vi "ReadUSB.vi"() -> ()   [LabVIEW 2018]
uses:
  <vilib>/Instr/_visa.llb/VISA Configure Serial Port (Instr).vi
panel:
  in  "ch":bool
  out "Erro de estado estacionário":dbl=3.0 format="%#_13g"
  out "Máximo Overshoot":dbl=3.0 format="%#_13g"
  out "Tempo de Subida":dbl=3.0 format="%#_13g"
  out "Tempo de Acomodação":dbl=3.0 format="%#_13g"
  in  "Modo Simulação":bool
  in  "Tempo de Simulação":dbl=3.0 format="%#_13g"
  out "cmd":T1(ring)
  in  "graph index":i32
  in  "Motor":cluster{"2":bool, "3":bool, "0":bool, "1":bool}={"2"=TRUE, "3"=FALSE, "0"=FALSE, "1"=FALSE}
  in  "Write":T2={"get_vel"=TRUE, "set_vel"=FALSE, "get PID cte"=FALSE, "set PID cte"=FALSE}
  out "String Enviada":string
  in  "kd":dbl format="%#_13g"
  in  "ki":dbl format="%#_13g"
  in  "kp":dbl format="%#_13g"
  in  "Vel":dbl format="%#_13g"
  out "kd":dbl
  out "ki":dbl
  out "kp":dbl
  out "String Tratada":string
  out "String Lida":string
  out "Vel":dbl
  in  "End":bool
  out "config error":errorcluster
  out "Vel":cluster{dbl, " Vel":dbl}(graph)
  in  "VISA resource name":refnum<visa-resource-name>
  # "APERTE END PARA ENCERRAR O PROGRAMA"
  # "VSS"
  # "SSL"
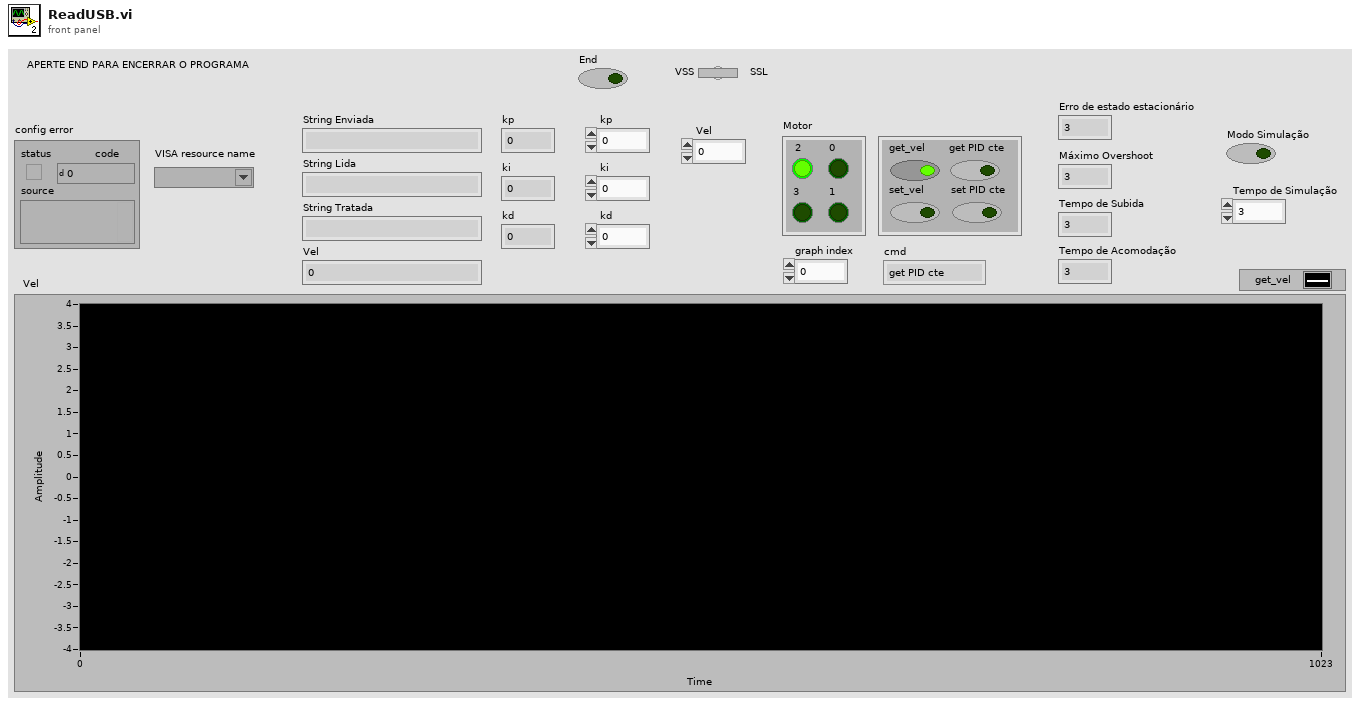
[diagram p1: front panel]
types:
  T1 = enum16{"get PID cte", "Set Vel", "Set PID cte", "get Vel"}
  T2 = cluster{"get_vel":bool, "set_vel":bool, "get PID cte":bool, "set PID cte":bool}
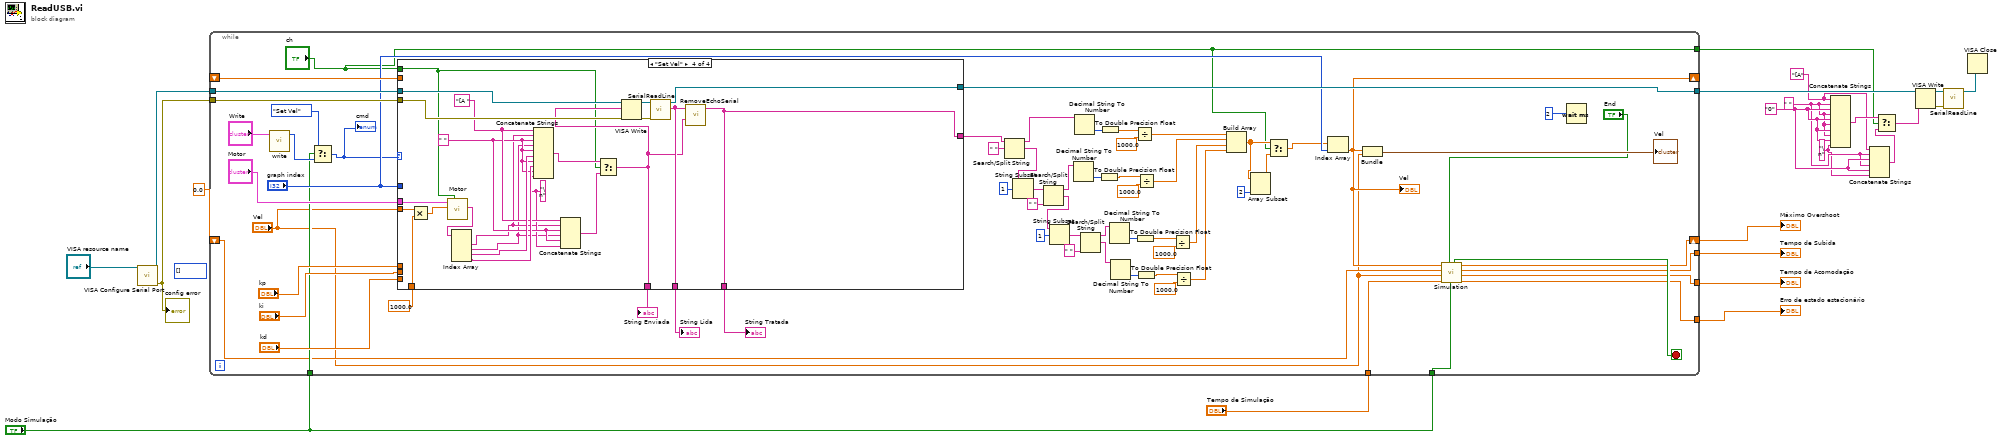
[diagram p0: block diagram]
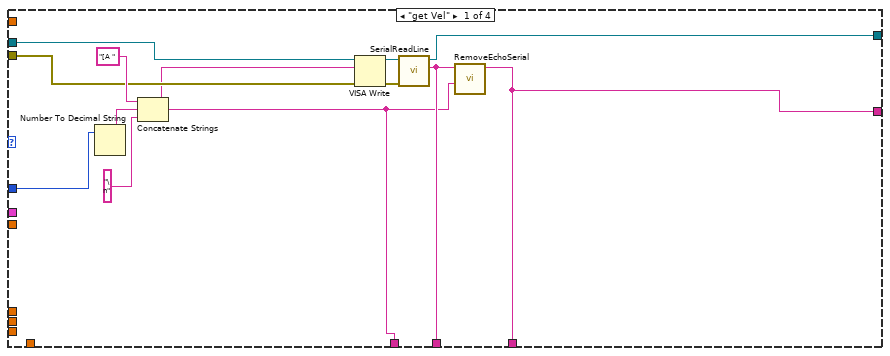
[diagram p2: hidden frame]
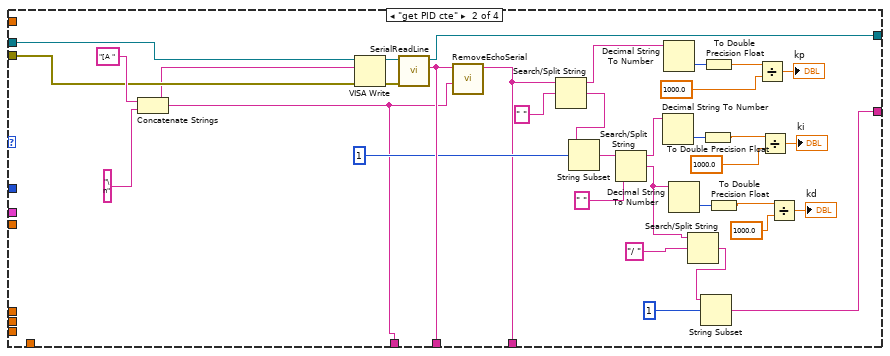
[diagram p3: hidden frame]
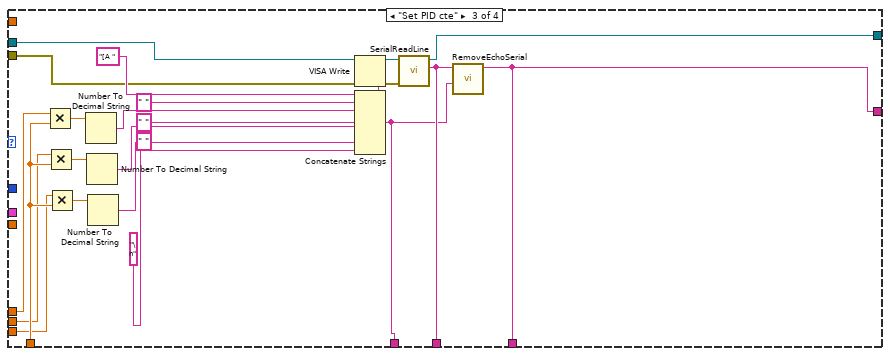
[diagram p4: hidden frame]
diagram:
  w2 = "\n" ("string")
  w4 = "0" ("string")
  w3 = " " ("string")
  w5 = "[A" ("write buffer")
  (unwired) i32[] []
  n1 = call-poly "VISA Configure Serial Port"("VISA resource name"="VISA resource name") -> ("VISA resource name out"=w20:refnum<visa-resource-name>, "error out"=w21:errorcluster)  [unwired: 13 in]
  "config error" <- w21
  n2 = while {
    tunnel: w21 -> [w87]
    tunnel: w20 -> [w86]
    tunnel: [w85] -> w16
    shift-right: [w31] -> _
    shift-left: _ -> [w82]
    tunnel: "Tempo de Simulação" -> [w42]
    tunnel: "Modo Simulação" -> [w39]
    tunnel: "Modo Simulação" -> [w37]
    shift-right: [w34] -> w12
    shift-left: 0.0 -> [w33]
    tunnel: [w32] -> w11
    tunnel: [w29] -> w10
    tunnel: [w28] -> w9
    tunnel: ["ch"] -> w7
    stop <- w40 stop-if-true
    n3 = call "write.vi"("Write"="Write") -> ("s? t:f"=w38:T1)  [unwired: 10 in]
    n4 = Select(t=T1."Set Vel", s=w37, f=w38) -> (s? t:f=w35:T1)
    "cmd" <- w35
    n5 = case shown="\"Set Vel\"" w35 {
      tunnel: w87 -> [w95 w129 w154 w178]
      tunnel: w86 -> [w94 w128 w153 w177]
      tunnel: [w93 w127 w152 w176] -> w85
      tunnel: "graph index" -> [w91 _ _ _]
      tunnel: [w92 w126 w151 w175] -> w84
      tunnel: [w90 w124 w136 w172] -> w83
      tunnel: w82 -> [_ _ _ _]
      tunnel: "Vel" -> [_ _ _ w174]
      tunnel: 1000.0 -> [_ _ w145 w173]
      tunnel: "kp" -> [_ _ w144 _]
      tunnel: "ki" -> [_ _ w143 _]
      tunnel: "kd" -> [_ _ w142 _]
      tunnel: [w90 w102 w136 w172] -> w48
      tunnel: [w89 w101 w135 w159] -> w47
      tunnel: "Motor" -> [_ _ _ w171]
      tunnel: "ch" -> [_ _ _ w158]
      frame "get Vel" {
        n6 = Number To Decimal String(number=w91) -> (decimal integer string=w100:string)  [unwired: 1 in]
        n7 = Concatenate Strings("[A " ("write buffer"), w100, "\n" ("string")) -> (w89:string)
        n8 = VISA Write(VISA resource name=w94, write buffer=w89, error in (no error)=w95) -> (VISA resource name out=w98:refnum<visa-resource-name>, error out=w99:errorcluster)  [unwired: 1 out]
        n9 = call "SerialReadLine.vi"("error in"=w99, "VISA resource name in"=w98) -> ("String"=w92:string, "VISA resource name out"=w93:refnum<visa-resource-name>)  [unwired: 7 in, 1 out]
        n10 = call "RemoveEchoSerial.vi"("message"=w89, "String in"=w92) -> ("String out"=w90:string)  [unwired: 9 in]
      }
      frame "get PID cte" {
        n11 = Concatenate Strings("[A " ("write buffer"), "\n" ("string")) -> (w101:string)
        n12 = VISA Write(VISA resource name=w128, write buffer=w101, error in (no error)=w129) -> (VISA resource name out=w132:refnum<visa-resource-name>, error out=w133:errorcluster)  [unwired: 1 out]
        n13 = call "SerialReadLine.vi"("error in"=w133, "VISA resource name in"=w132) -> ("String"=w126:string, "VISA resource name out"=w127:refnum<visa-resource-name>)  [unwired: 7 in, 1 out]
        n14 = call "RemoveEchoSerial.vi"("message"=w101, "String in"=w126) -> ("String out"=w124:string)  [unwired: 9 in]
        n15 = Search/Split String(string=w124, search string/char (-)=" ") -> (substring before match=w123:string, match + rest of string=w120:string)  [unwired: 1 in, 1 out]
        n16 = String Subset(string=w120, offset (0)=1) -> (substring=w119:string)  [unwired: 1 in]
        n17 = Search/Split String(string=w119, search string/char (-)=" ") -> (substring before match=w116:string, match + rest of string=w104:string)  [unwired: 1 in, 1 out]
        n18 = Decimal String To Number(string=w116) -> (number=w121:i32)  [unwired: 2 in, 1 out]
        n19 = Decimal String To Number(string=w123) -> (number=w134:i32)  [unwired: 2 in, 1 out]
        n20 = Decimal String To Number(string=w104) -> (number=w117:i32)  [unwired: 2 in, 1 out]
        n21 = Search/Split String(string=w104, search string/char (-)="/ ") -> (match + rest of string=w103:string)  [unwired: 1 in, 2 out]
        n22 = String Subset(string=w103, offset (0)=1) -> (substring=w102:string)  [unwired: 1 in]
        n23 = To Double Precision Float(number=w121) -> (double precision float=w108:dbl)
        n24 = To Double Precision Float(number=w134) -> (double precision float=w115:dbl)
        n25 = To Double Precision Float(number=w117) -> (double precision float=w107:dbl)
        n26 = Divide(x=w115, y=1000.0) -> (x/y=→"kp":dbl)
        n27 = Divide(x=w108, y=1000.0) -> (x/y=→"ki":dbl)
        n28 = Divide(x=w107, y=1000.0) -> (x/y=→"kd":dbl)
      }
      frame "Set PID cte" {
        n29 = Multiply(x=w144, y=w145) -> (x*y=w150:dbl)
        n30 = Multiply(x=w143, y=w145) -> (x*y=w149:dbl)
        n31 = Multiply(x=w142, y=w145) -> (x*y=w148:dbl)
        n32 = Number To Decimal String(number=w150) -> (decimal integer string=w141:string)  [unwired: 1 in]
        n33 = Number To Decimal String(number=w149) -> (decimal integer string=w147:string)  [unwired: 1 in]
        n34 = Number To Decimal String(number=w148) -> (decimal integer string=w140:string)  [unwired: 1 in]
        n35 = Concatenate Strings("[A " ("write buffer"), " " ("string"), w141, " " ("string"), w147, " " ("string"), w140, "\n" ("string")) -> (w135:string)
        n36 = VISA Write(VISA resource name=w153, write buffer=w135, error in (no error)=w154) -> (VISA resource name out=w156:refnum<visa-resource-name>, error out=w157:errorcluster)  [unwired: 1 out]
        n37 = call "SerialReadLine.vi"("error in"=w157, "VISA resource name in"=w156) -> ("String"=w151:string, "VISA resource name out"=w152:refnum<visa-resource-name>)  [unwired: 7 in, 1 out]
        n38 = call "RemoveEchoSerial.vi"("message"=w135, "String in"=w151) -> ("String out"=w136:string)  [unwired: 9 in]
      }
      frame "Set Vel" {
        w165 = " " ("string")
        w164 = "\n" ("string")
        w166 = "[A " ("write buffer")
        n39 = Multiply(x=w174, y=w173) -> (x*y=w170:dbl)
        n40 = call "Motor.vi"("Boolean"=w158, "vel"=w170, "Motor"=w171) -> ("appended array"=w169:string[])  [unwired: 8 in]
        n41 = Index Array(array=w169) -> (element #1=w163:string, element #2=w162:string, element #3=w168:string, element #4=w167:string)  [unwired: 4 in]
        n42 = Concatenate Strings(w166, w163, w165, w162, w165, w168, w165, w167, w165, w164) -> (w161:string)
        n43 = Concatenate Strings(w166, w163, w165, w162, w165, w164) -> (w160:string)
        n44 = Select(t=w161, s=w158, f=w160) -> (s? t:f=w159:string)
        n45 = VISA Write(VISA resource name=w177, write buffer=w159, error in (no error)=w178) -> (VISA resource name out=w179:refnum<visa-resource-name>, error out=w180:errorcluster)  [unwired: 1 out]
        n46 = call "SerialReadLine.vi"("error in"=w180, "VISA resource name in"=w179) -> ("String"=w175:string, "VISA resource name out"=w176:refnum<visa-resource-name>)  [unwired: 7 in, 1 out]
        n47 = call "RemoveEchoSerial.vi"("message"=w159, "String in"=w175) -> ("String out"=w172:string)  [unwired: 9 in]
      }
    }
    "String Lida" <- w84
    "String Tratada" <- w83
    "String Enviada" <- w47
    n48 = Search/Split String(string=w48, search string/char (-)=" ") -> (substring before match=w75:string, match + rest of string=w72:string)  [unwired: 1 in, 1 out]
    n49 = String Subset(string=w72, offset (0)=1) -> (substring=w71:string)  [unwired: 1 in]
    n50 = Search/Split String(string=w71, search string/char (-)=" ") -> (substring before match=w69:string, match + rest of string=w61:string)  [unwired: 1 in, 1 out]
    n51 = String Subset(string=w61, offset (0)=1) -> (substring=w63:string)  [unwired: 1 in]
    n52 = Decimal String To Number(string=w69) -> (number=w73:i32)  [unwired: 2 in, 1 out]
    n53 = Decimal String To Number(string=w75) -> (number=w77:i32)  [unwired: 2 in, 1 out]
    n54 = Search/Split String(string=w63, search string/char (-)=" ") -> (substring before match=w57:string, match + rest of string=w53:string)  [unwired: 1 in, 1 out]
    n55 = To Double Precision Float(number=w73) -> (double precision float=w65:dbl)
    n56 = To Double Precision Float(number=w77) -> (double precision float=w68:dbl)
    n57 = Decimal String To Number(string=w57) -> (number=w58:i32)  [unwired: 2 in, 1 out]
    n58 = Decimal String To Number(string=w53) -> (number=w56:i32)  [unwired: 2 in, 1 out]
    n59 = Divide(x=w68, y=1000.0) -> (x/y=w52:dbl)
    n60 = To Double Precision Float(number=w58) -> (double precision float=w60:dbl)
    n61 = Divide(x=w65, y=1000.0) -> (x/y=w51:dbl)
    n62 = To Double Precision Float(number=w56) -> (double precision float=w54:dbl)
    n63 = Divide(x=w60, y=1000.0) -> (x/y=w50:dbl)
    n64 = Divide(x=w54, y=1000.0) -> (x/y=w49:dbl)
    n65 = Build Array(w52, w51, w50, w49) -> (w26:dbl[])
    n66 = Array Subset(array=w26, length=2) -> (w25:dbl[])  [unwired: 1 in]
    n67 = Select(t=w26, s="ch", f=w25) -> (s? t:f=w27:dbl[])
    n68 = Index Array(array=w27, index="graph index") -> (element=w31:dbl)
    "Vel" <- w31
    n69 = Bundle(w31, "Vel"="Vel") -> (→"Vel":cluster{dbl, " Vel":dbl})  [unwired: 1 in]
    n70 = call "Simulation.vi"("Modo Simulação"=w39, "Tempo de Simulação"=w42, "End"="End", "set_vel"="Vel", "Mp"=w33, "read_vel"=w31) -> ("erro de estado estacionário"=w28:dbl, "Tempo de acomodação"=w29:dbl, "Tempo de subida"=w32:dbl, "Máximo Overshoot"=w34:dbl, "Boolean"=w40:bool)  [unwired: 1 in]
    n71 = Wait (ms)(milliseconds to wait=u32 2) -> ()  [unwired: 1 out]
  }
  "Tempo de Acomodação" <- w10
  "Tempo de Subida" <- w11
  "Máximo Overshoot" <- w12
  "Erro de estado estacionário" <- w9
  n72 = Concatenate Strings(w5, w3, w4, w3, w4, w3, w4, w3, w4, w2) -> (w8:string)
  n73 = Concatenate Strings(w5, w3, w4, w3, w4, w2) -> (w1:string)
  n74 = Select(t=w8, s=w7, f=w1) -> (s? t:f=w6:string)
  n75 = VISA Write(VISA resource name=w16, write buffer=w6) -> (VISA resource name out=w18:refnum<visa-resource-name>, error out=w19:errorcluster)  [unwired: 1 in, 1 out]
  n76 = call "SerialReadLine.vi"("error in"=w19, "VISA resource name in"=w18) -> ("VISA resource name out"=w17:refnum<visa-resource-name>)  [unwired: 7 in, 2 out]
  n77 = VISA Close(VISA resource name=w17) -> ()  [unwired: 1 in, 1 out]
